vi "Simulator.vi"() -> ()   [LabVIEW 2017]
uses:
  <vilib>/Utility/file.llb/Write Delimited Spreadsheet (DBL).vi
  <vilib>/Utility/file.llb/Write Delimited Spreadsheet (string).vi
panel:
  in  "File Path Control":path
  in  "delta(ms)":i32
  in  "Off Time(ms)":i32
  in  "No of Rotation":i32
  in  "Dwell Time(ms)":i32
  out "Square":waveform(dbl)[](graph)
  in  "Frequency(Hz)":dbl=20.0 caption="Frequency"
  in  "Duty Cycle (%)":dbl=50.0
  # "Signal Generator"
  # "Test Properties"
  # "Signal Properties"
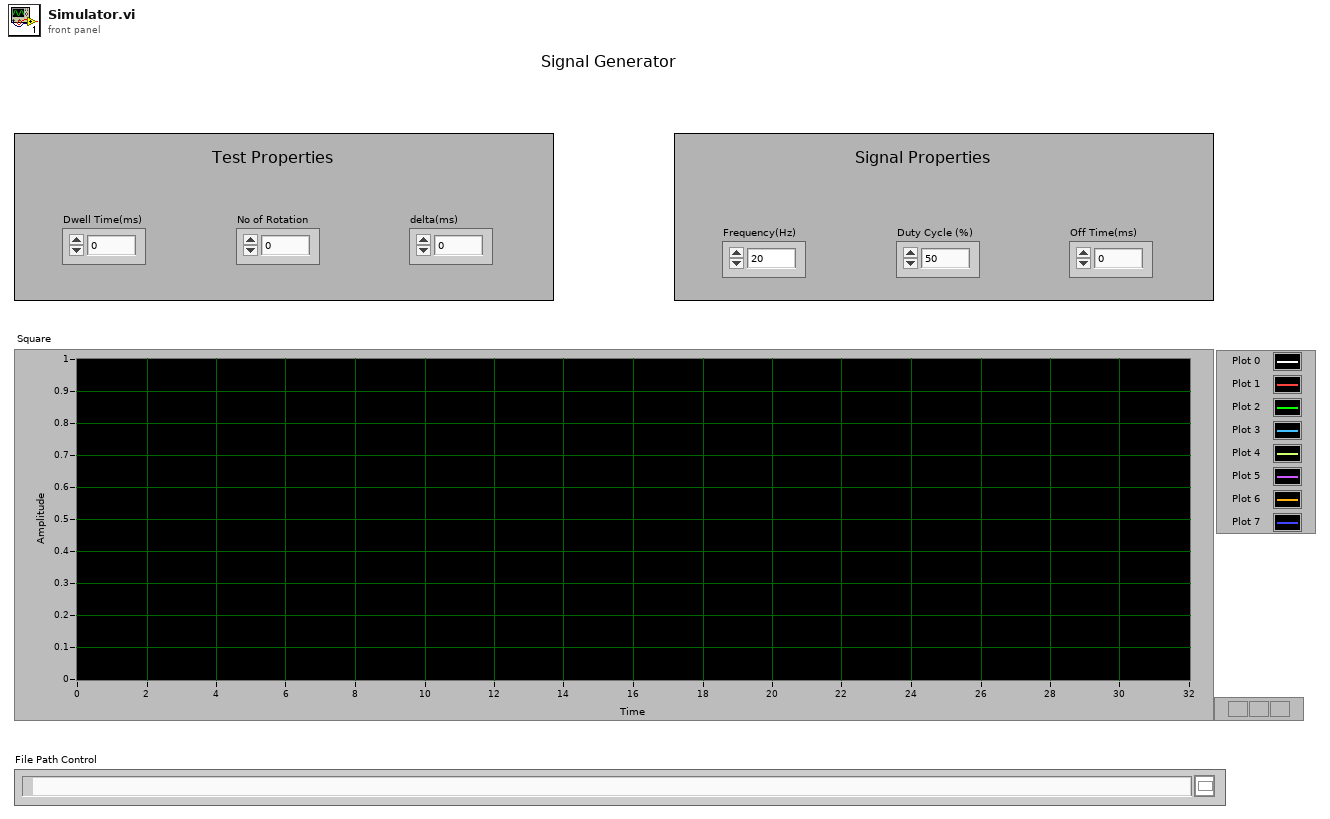
[diagram p1: front panel]
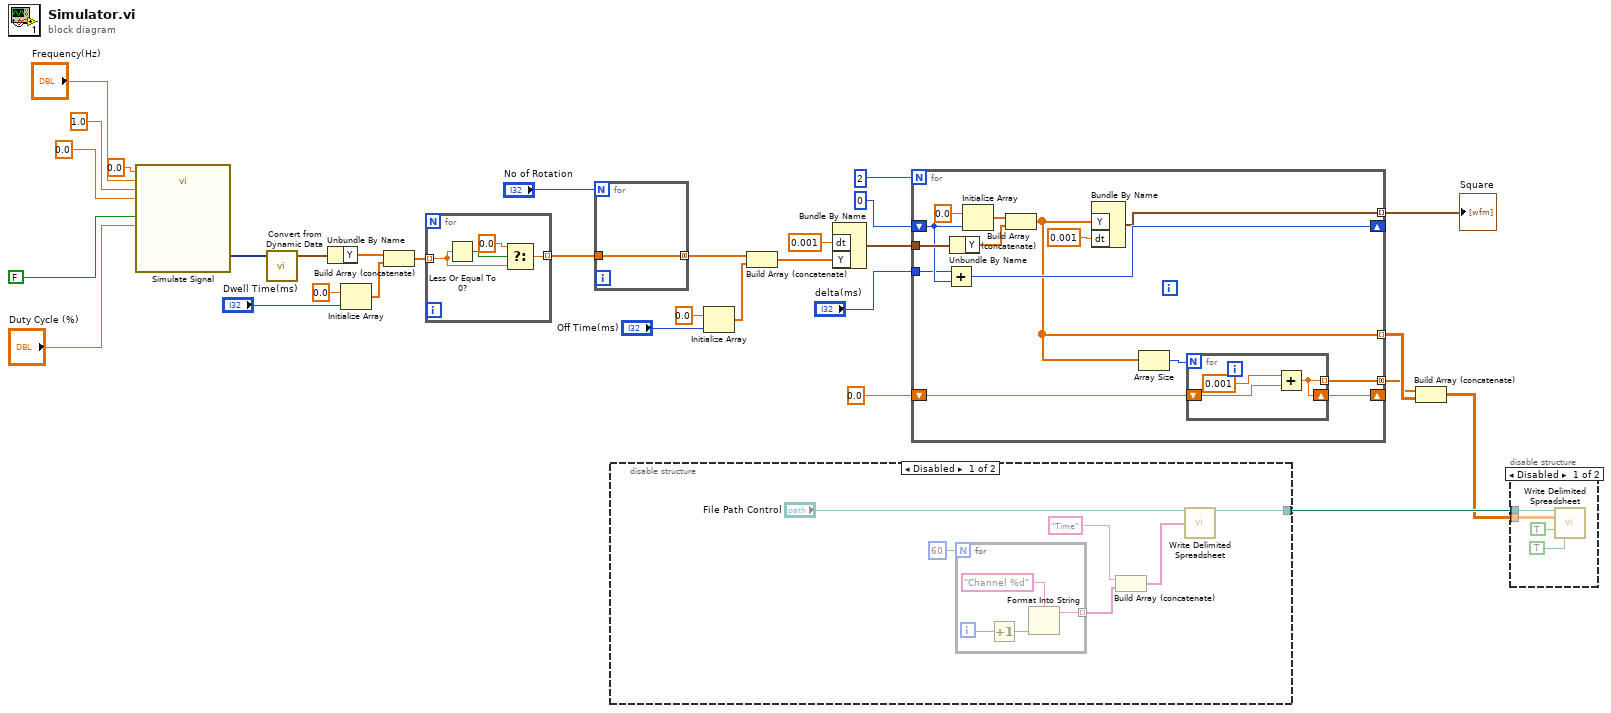
[diagram p0: block diagram]
diagram:
  n1 = call "Simulate Signal"("Offset"=0.0, "Duty Cycle (%)"="Duty Cycle (%)", "Reset Signal"=FALSE, "Frequency"="Frequency(Hz)", "Amplitude"=1.0, "Phase"=0.0) -> ("Square"=w25:dynamicdata)  [unwired: 8 in, 1 out]
  n2 = call "Convert from Dynamic Data"("Dynamic Data Type"=w25) -> ("Waveform"=w21:waveform(dbl))  [unwired: 3 in]
  n3 = Unbundle By Name(w21) -> ("Y"=w20:dbl[])
  n4 = Initialize Array(0.0 ("element"), "Dwell Time(ms)") -> (w19:dbl[])
  n5 = Build Array (concatenate)(w20, w19) -> (w17:dbl[])
  n6 = for {
    tunnel: w17 -> [w33] mode=indexing
    tunnel: [w32] -> w16 mode=indexing
    n7 = Less Or Equal To 0?(x=w33) -> (x <= 0?=w35:bool)
    n8 = Select(t=0.0, s=w35, f=w33) -> (s? t:f=w32:dbl)
  }
  n9 = for {
    N: "No of Rotation" -> [_]
    tunnel: w16 -> [w36]
    tunnel: [w36] -> w13 mode=concatenating
  }
  n10 = disable-structure shown="Disabled" {
    disable-tunnel: [w41 _] -> w5
    frame Disabled {
      n11 = for {
        N: 60 -> [_]
        tunnel: [w43] -> w38 mode=indexing
        i -> [w44]
        n12 = Increment(x=w44) -> (x+1=w45:i32)
        n13 = Format Into String(format string="Channel %d", w45) -> (resulting string=w43:string)  [unwired: 2 in, 1 out]
      }
      n14 = Build Array (concatenate)("Time", w38) -> (w37:string[])
      n15 = call-poly <vilib>:"Write Delimited Spreadsheet.vi"("file path (dialog if empty)"="File Path Control", "1D data"=w37) -> ("new file path (Not A Path if cancelled)"=w41:path)  [unwired: 12 in, 1 out]
    }
    frame Enabled {
    }
  }
  n16 = Initialize Array(0.0 ("element"), "Off Time(ms)") -> (w12:dbl[])
  n17 = Build Array (concatenate)(w13, w12) -> (w11:dbl[])
  n18 = Bundle By Name("dt"=0.001, "Y"=w11) -> (w9:waveform(dbl))  [unwired: 1 in]
  n19 = for {
    N: 2 -> [_]
    tunnel: w9 -> [w60]
    shift-right: [w56] -> _
    shift-left: 0 -> [w58]
    tunnel: "delta(ms)" -> [w57]
    tunnel: [w53] -> w6 mode=indexing
    tunnel: [w50] -> w4 mode=indexing
    tunnel: [w49] -> w3 mode=concatenating
    shift-right: [w47] -> _
    shift-left: 0.0 ("dt") -> [w48]
    n20 = Add(x=w57, y=w58) -> (x+y=w56:i32)
    n21 = Unbundle By Name(w60) -> ("Y"=w55:dbl[])
    n22 = Initialize Array(0.0 ("element"), w58) -> (w54:dbl[])
    n23 = Build Array (concatenate)(w54, w55) -> (w50:dbl[])
    n24 = Bundle By Name("Y"=w50, "dt"=0.001) -> (w53:waveform(dbl))  [unwired: 1 in]
    n25 = Array Size(array=w50) -> (size(s)=w51:i32)
    n26 = for {
      N: w51 -> [_]
      tunnel: [w62] -> w49 mode=indexing
      shift-right: [w62] -> w47
      shift-left: w48 -> [w63]
      n27 = Add(x=0.001 ("dt"), y=w63) -> (x+y=w62:dbl)
    }
  }
  "Square" <- w6
  n28 = Build Array (concatenate)(w3, w4) -> (w2:dbl[][])
  n29 = disable-structure shown="Disabled" {
    disable-tunnel: w5 -> [w67 _]
    disable-tunnel: w2 -> [w64 _]
    frame Disabled {
      n30 = call-poly <vilib>:"Write Delimited Spreadsheet.vi"("file path (dialog if empty)"=w67, "2D data"=w64, "append to file? (new file:F)"=TRUE, "transpose? (no:F)"=TRUE) -> ()  [unwired: 10 in, 2 out]
    }
    frame Enabled {
    }
  }
